vi "main.vi"(11 "lv_Numeric":i32) -> (3 "lv_String":string)   [LabVIEW 2018]
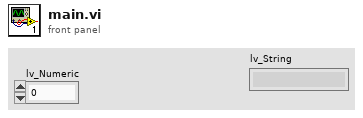
[diagram p1: front panel]
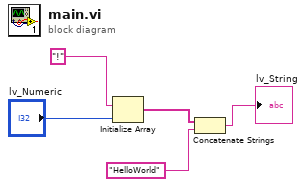
[diagram p0: block diagram]
diagram:
  n1 = Initialize Array("!", "lv_Numeric") -> (w2:string[])
  n2 = Concatenate Strings(w2, "HelloWorld") -> (→"lv_String":string)
